vi "PowerOFF.vi"(8 "error in (no error)":errorcluster, 11 "CDPlayer in":refnum<class "CDPlayer.lvclass">) -> (0 "error out":errorcluster, 2 "Message":string, 3 "CDPlayer out":refnum<class "CDPlayer.lvclass">)   [LabVIEW 2013, in "CDPlayer.lvclass"]
uses:
  CDPlayer.lvclass
  CDPlayer.lvclass/CDPlayer.ctl
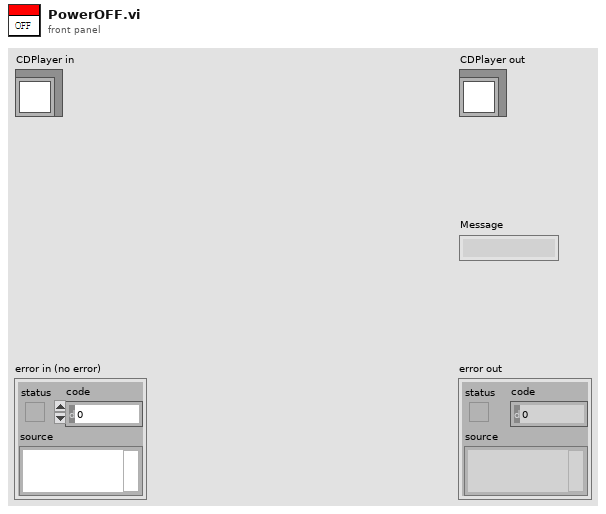
[diagram p1: front panel]
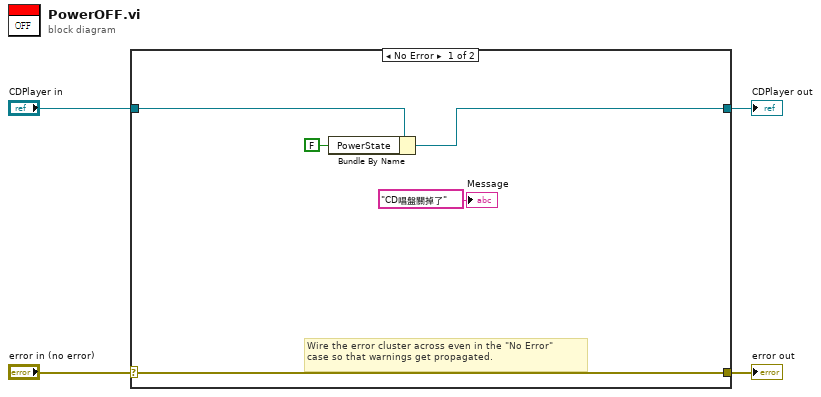
[diagram p0: block diagram]
diagram:
  n1 = case shown="No Error" "error in (no error)" {
    selector: "error in (no error)" -> [w9 w11]
    tunnel: [w9 w11] -> w3
    tunnel: [w6 w10] -> w1
    tunnel: "CDPlayer in" -> [w7 w10]
    frame No Error {
      # "Wire the error cluster across even in the \"No Error\"\ncase so that warnings get propagated."
      n2 = Bundle By Name(cluster=w7, "PowerState"=FALSE) -> (w6:refnum<class "CDPlayer.lvclass">)
      "Message" <- "CD唱盤關掉了" ("Message")
    }
    frame Error {
    }
  }
  "error out" <- w3
  "CDPlayer out" <- w1
